vi "fpga_Channel_fifo.vi"(2 "ID":u8, 3 "Signal IN":bool, 4 "Schedule":u8, 5 "Main clock":u32) -> (0 "Data Available":bool, 1 "32 bit Output":u32)   [LabVIEW 2011]
uses:
  <vilib>/rvi/DataTransferAndStorage/Container/Common/niFpgaContainerMetaDataKey.ctl
  <vilib>/rvi/DataTransferAndStorage/Container/Common/niFpgaContainerState.ctl
  <vilib>/rvi/DataTransferAndStorage/Container/Common/niFpgaDataTypeControl.ctl
  <vilib>/rvi/DataTransferAndStorage/Container/Common/niFpgaContainerImplementationControl.ctl
  <vilib>/rvi/DataTransferAndStorage/Container/Common/niFpgaContainerArbitrationOptionsControl.ctl
  <vilib>/rvi/DataTransferAndStorage/Container/Common/niFpgaTransferTypeControl.ctl
  <vilib>/rvi/DataTransferAndStorage/Container/Common/niFpgaContainerInitializationParameters.ctl
  <vilib>/rvi/Memory/Memory_Types/niFpgaMemoryInterfaceConfiguration.ctl
  <vilib>/rvi/FIFO/Fifo_Types/niFpgaFifoControlLogicControl.ctl
  <vilib>/rvi/eio/common/nirviEmuReportErrorAndStop.vi
  <vilib>/rvi/DataTransferAndStorage/Container/Common/niFpgaContainerSetEmuInfo.vi
  <vilib>/rvi/DataTransferAndStorage/Container/Common/niFpgaContainerGetUniqueNameForEmu.vi
  <vilib>/rvi/FIFO/Fifo_Resource/nirvififoEmulationSetSize.vi
  <vilib>/rvi/LocalResourceManager/LocalResourceManager.xnode
  <vilib>/rvi/DataTransferAndStorage/Container/XNode/niFpgaContainer.xnode
  <vilib>/rvi/FIFO/Fifo_Resource/nirvififoEmulationWrite.vi
  <vilib>/rvi/FIFO/Fifo_Resource/nirvififoEmulationRead.vi
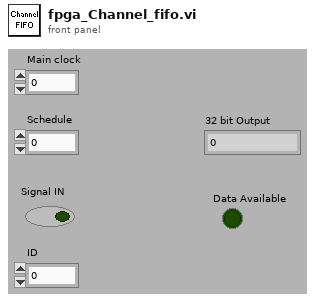
[diagram p1: front panel]
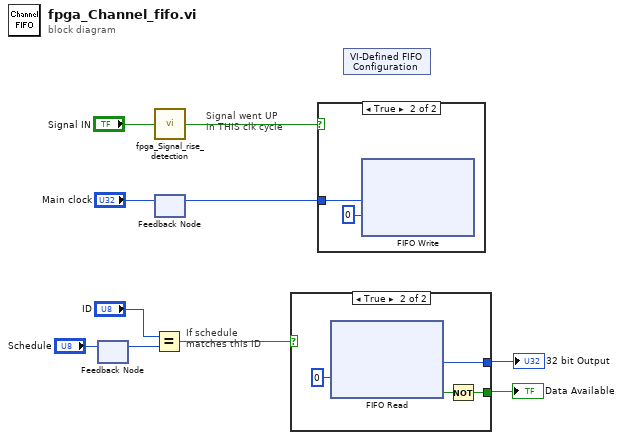
[diagram p0: block diagram]
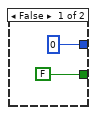
[diagram p2: hidden frame]
diagram:
  # "If schedule \nmatches this ID"
  # "Signal went UP\nin THIS clk cycle"
  n1 = feedback-in #1("Schedule") -> ()
  n2 = feedback #1() -> (w1:u8)  [unwired: 1 in]
  n3 = Equal?(x="ID", y=w1) -> (x = y?=w3:bool)
  n4 = call "fpga_Signal_rise_detection.vi"("Signal IN"="Signal IN") -> ("Signal change LOW->HIGH?"=w4:bool)
  n5 = feedback-in #2("Main clock") -> ()
  n6 = feedback #2() -> (w2:u32)  [unwired: 1 in]
  n7 = case shown="True" w3 {
    tunnel: [FALSE w13] -> w8
    tunnel: [u32 0 ("Element") w14] -> w9
    frame False {
    }
    frame True {
      n8 = xnode ("FIFO Read")("Timeout"=0) -> ("Element"=w14:u32, "Timed Out?"=w15:bool)  [unwired: 1 in, 1 out]
      n9 = Not(x=w15) -> (.not. x?=w13:bool)
    }
  }
  "32 bit Output" <- w9
  "Data Available" <- w8
  n10 = case shown="True" w4 {
    tunnel: w2 -> [_ w17]
    frame False {
    }
    frame True {
      n11 = xnode ("FIFO Write")("Element"=w17, "Timeout"=0) -> ()  [unwired: 1 in, 2 out]
    }
  }
  n12 = xnode "VI-Defined FIFO Configuration"() -> ()  [unwired: 1 out]
